vi "stringArray.vi"(11 "CNC strings":string) -> (3 "stringArray":string[](array[string]))   [LabVIEW 2019]
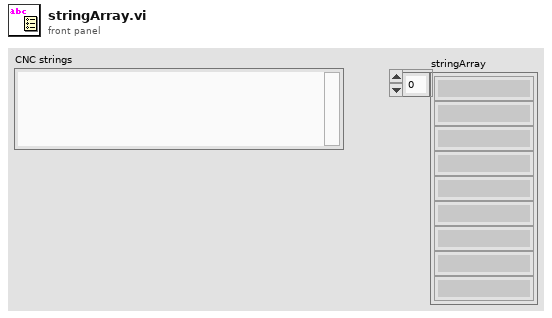
[diagram p1: front panel]
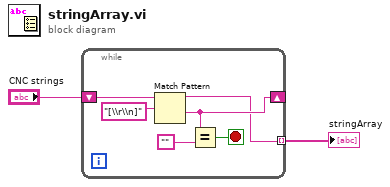
[diagram p0: block diagram]
diagram:
  n1 = while {
    shift-right: [w6] -> _
    shift-left: "CNC strings" -> [w8]
    tunnel: [w3] -> w1 mode=indexing
    stop <- w4 stop-if-true
    n2 = Match Pattern(string=w8, regular expression="[\\r\\n]") -> (before substring=w3:string, after substring=w6:string)  [unwired: 1 in, 2 out]
    n3 = Equal?(x=w6, y="") -> (x = y?=w4:bool)
  }
  "stringArray" <- w1
